vi "Excel___Adjust Main Page.vi"(0 "Cells Ref In":refnum<k7>, 1 "Standards Used":string[][](array[string]), 2 "Standards Count":i32, 3 "Machine Specs":string[][](array[string]), 4 "Specs Count":i32, 5 "Error In":errorcluster, 9 "Too Many?":bool) -> (14 "Cells Ref Out":refnum<k7>, 19 "Error Out":errorcluster)   [LabVIEW 2013]
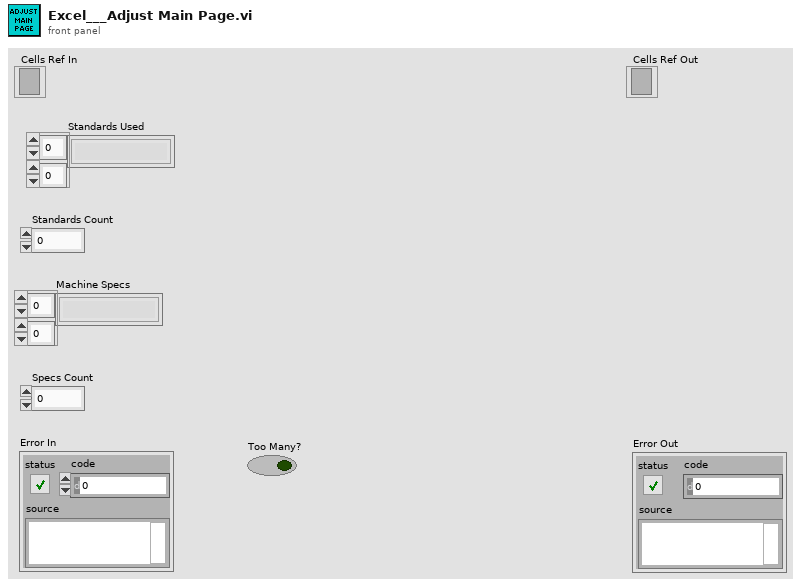
[diagram p1: front panel]
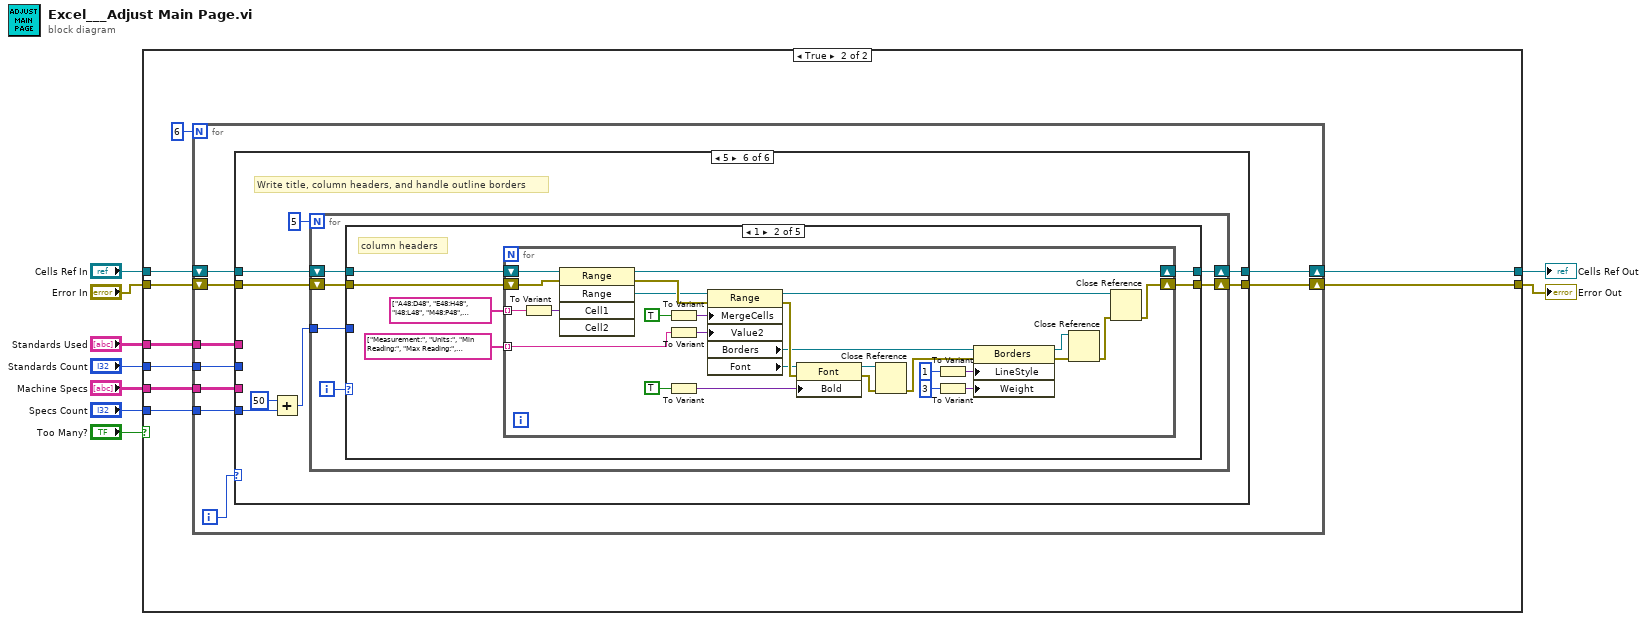
[diagram p0: block diagram]
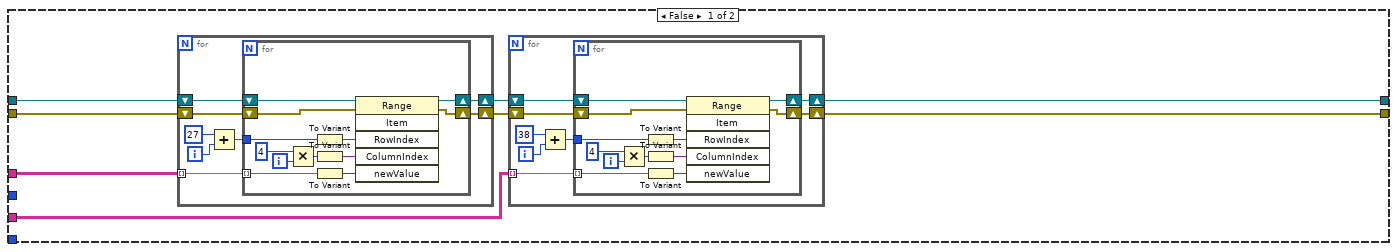
[diagram p2: hidden frame]
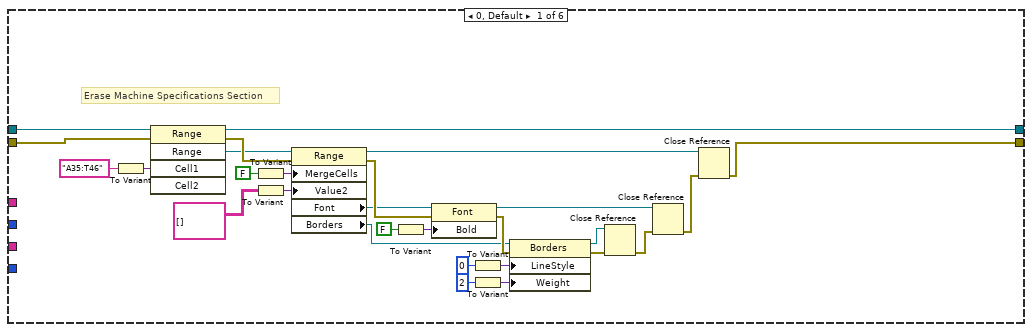
[diagram p3: hidden frame]
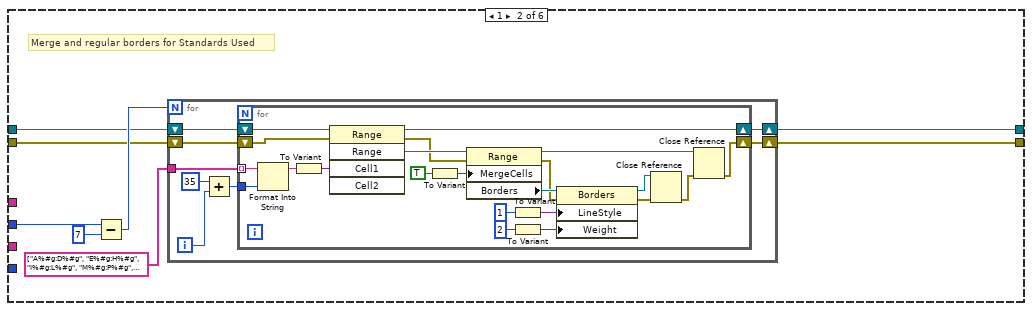
[diagram p4: hidden frame]
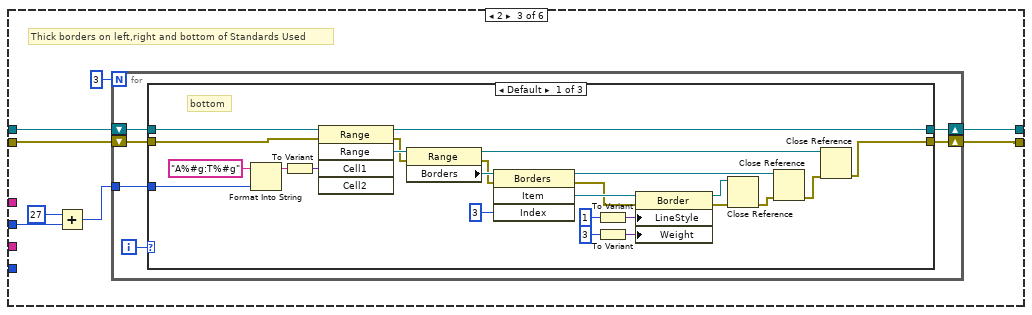
[diagram p5: hidden frame]
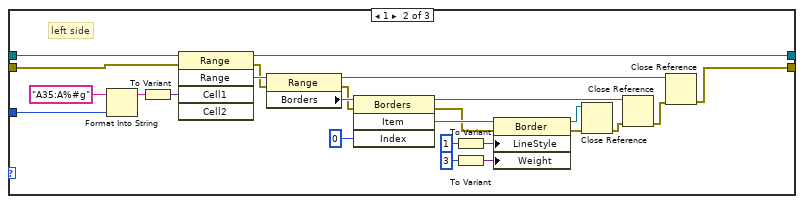
[diagram p6: hidden frame]
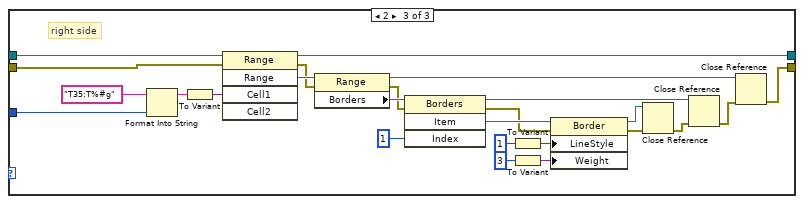
[diagram p7: hidden frame]
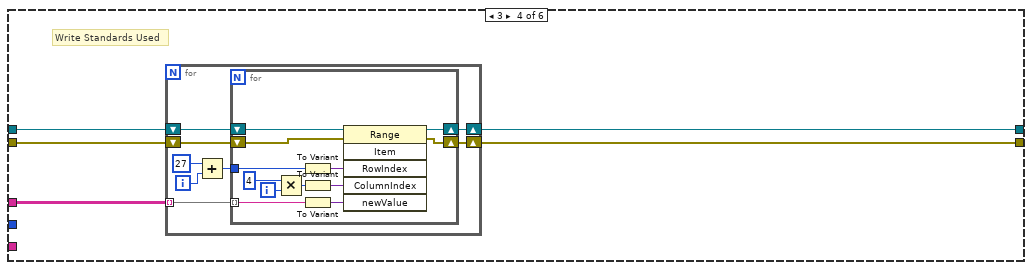
[diagram p8: hidden frame]
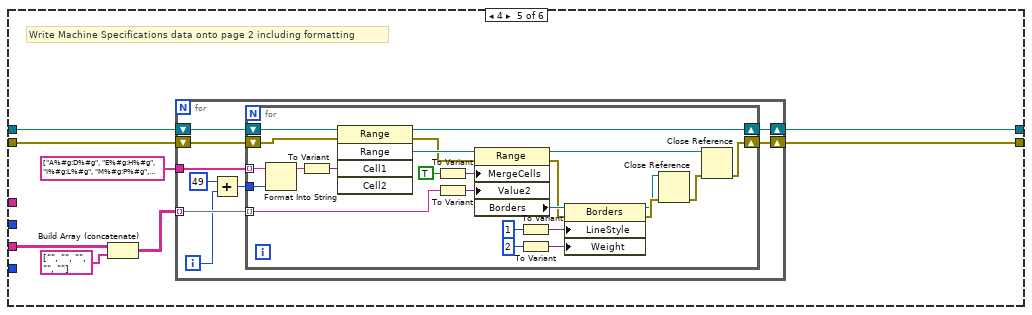
[diagram p9: hidden frame]
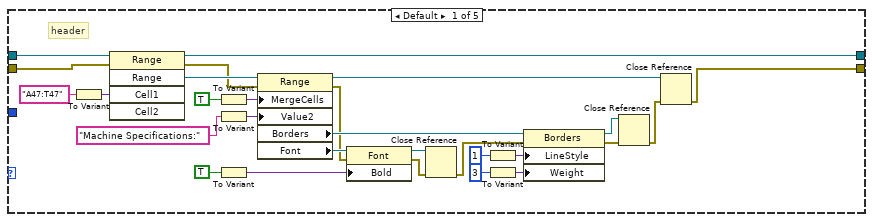
[diagram p10: hidden frame]
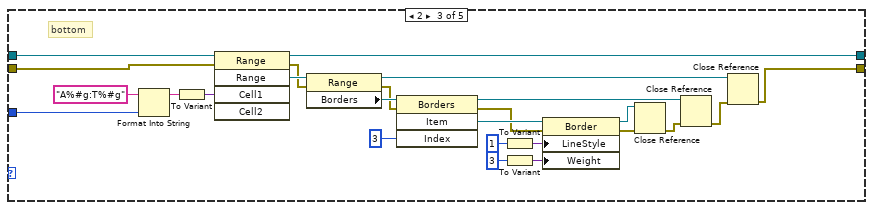
[diagram p11: hidden frame]
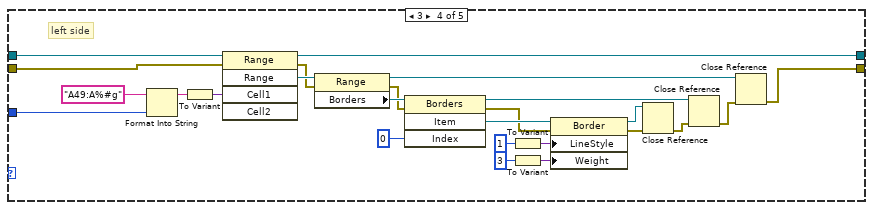
[diagram p12: hidden frame]
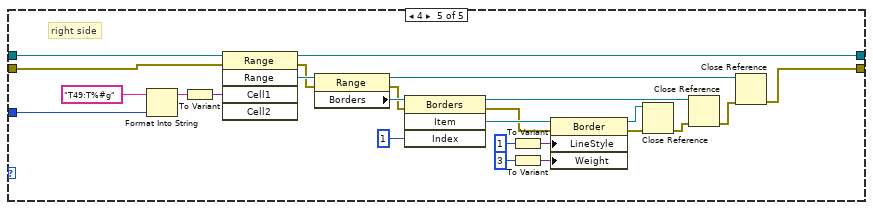
[diagram p13: hidden frame]
diagram:
  n1 = case shown="True" "Too Many?" {
    tunnel: "Error In" -> [w17 w65]
    tunnel: "Standards Used" -> [w16 w64]
    tunnel: "Cells Ref In" -> [w14 w66]
    tunnel: [w13 w61] -> w4
    tunnel: [w12 w62] -> w3
    tunnel: "Machine Specs" -> [w10 w63]
    tunnel: "Standards Count" -> [_ w60]
    tunnel: "Specs Count" -> [_ w59]
    frame False {
      n2 = for {
        shift-right: [w23] -> w11
        shift-left: w14 -> [w25]
        shift-right: [w22] -> w15
        shift-left: w17 -> [w24]
        tunnel: w16 -> [w21] mode=indexing
        i -> [w20]
        n3 = Add(x=27, y=w20) -> (x+y=w18:i32)
        n4 = for {
          shift-right: [w35] -> w23
          shift-left: w25 -> [w37]
          shift-right: [w32] -> w22
          shift-left: w24 -> [w36]
          tunnel: w21 -> [w34] mode=indexing
          tunnel: w18 -> [w29]
          i -> [w28]
          n5 = Multiply(x=4, y=w28) -> (x*y=w26:i32)
          n6 = To Variant(anything=w29) -> (Variant=w31:variant)
          n7 = To Variant(anything=w26) -> (Variant=w30:variant)
          n8 = To Variant(anything=w34) -> (Variant=w33:variant)
          n9 = invoke class="Range" method="Item"(reference=w37, error in=w36, "RowIndex"=w31, "ColumnIndex"=w30, "newValue"=w33) -> (reference out=w35:refnum<k7>, error out=w32:errorcluster)  [unwired: 1 in, 4 out]
        }
      }
      n10 = for {
        shift-right: [w43] -> w13
        shift-left: w11 -> [w45]
        shift-right: [w42] -> w12
        shift-left: w15 -> [w44]
        tunnel: w10 -> [w41] mode=indexing
        i -> [w40]
        n11 = Add(x=38, y=w40) -> (x+y=w38:i32)
        n12 = for {
          shift-right: [w55] -> w43
          shift-left: w45 -> [w57]
          shift-right: [w52] -> w42
          shift-left: w44 -> [w56]
          tunnel: w41 -> [w54] mode=indexing
          tunnel: w38 -> [w49]
          i -> [w48]
          n13 = Multiply(x=4, y=w48) -> (x*y=w46:i32)
          n14 = To Variant(anything=w49) -> (Variant=w51:variant)
          n15 = To Variant(anything=w46) -> (Variant=w50:variant)
          n16 = To Variant(anything=w54) -> (Variant=w53:variant)
          n17 = invoke class="Range" method="Item"(reference=w57, error in=w56, "RowIndex"=w51, "ColumnIndex"=w50, "newValue"=w53) -> (reference out=w55:refnum<k7>, error out=w52:errorcluster)  [unwired: 1 in, 4 out]
        }
      }
    }
    frame True {
      n18 = for {
        N: 6 -> [_]
        tunnel: w64 -> [w73]
        tunnel: w63 -> [w72]
        shift-right: [w70] -> w61
        shift-left: w66 -> [w75]
        shift-right: [w71] -> w62
        shift-left: w65 -> [w74]
        tunnel: w60 -> [w68]
        tunnel: w59 -> [w67]
        i -> [w69]
        n19 = case shown="5" w69 {
          tunnel: w75 -> [w79 w107 w149 w235 w262 w303]
          tunnel: w74 -> [w78 w106 w148 w234 w261 w302]
          tunnel: w73 -> [_ _ _ w233 _ _]
          tunnel: w72 -> [_ _ _ _ w260 _]
          tunnel: [w77 w105 w146 w232 w257 w301] -> w70
          tunnel: [w76 w104 w145 w231 w256 w300] -> w71
          tunnel: w68 -> [_ w110 w144 _ _ _]
          tunnel: w67 -> [_ _ _ _ _ w299]
          frame 0, Default {
            # "Erase Machine Specifications Section"
            n20 = To Variant(anything="A35:T46") -> (Variant=w80:variant)
            n21 = invoke class="Range" method="Range"(reference=w79, error in=w78, "Cell1"=w80) -> (reference out=w77:refnum<k7>, error out=w96:errorcluster, "Range"=w82:refnum<k7>)  [unwired: 2 in, 2 out]
            n22 = To Variant(anything=FALSE) -> (Variant=w83:variant)
            n23 = To Variant(anything=string[][] []) -> (Variant=w86:variant)
            n24 = property class="Range"(reference=w82, error in=w96, "MergeCells"=w83, "Value2"=w86) -> (reference out=w102:refnum<k7>, error out=w97:errorcluster, "Font"=w85:refnum<k7>, "Borders"=w88:refnum<k7>)
            n25 = To Variant(anything=FALSE) -> (Variant=w94:variant)
            n26 = property class="Font"(reference=w85, error in=w97, "Bold"=w94) -> (reference out=w101:refnum<k7>, error out=w95:errorcluster)
            n27 = To Variant(anything=0) -> (Variant=w89:variant)
            n28 = To Variant(anything=2) -> (Variant=w90:variant)
            n29 = property class="Borders"(reference=w88, error in=w95, "LineStyle"=w89, "Weight"=w90) -> (reference out=w99:refnum<k7>, error out=w98:errorcluster)
            n30 = Close Reference(reference=w99, error in (no error)=w98) -> (error out=w100:errorcluster)
            n31 = Close Reference(reference=w101, error in (no error)=w100) -> (error out=w103:errorcluster)
            n32 = Close Reference(reference=w102, error in (no error)=w103) -> (error out=w76:errorcluster)
          }
          frame 1 {
            # "Merge and regular borders for Standards Used"
            n33 = Subtract(x=w110, y=7) -> (x-y=w108:i32)
            n34 = for {
              N: w108 -> [_]
              tunnel: string[] ["A%#g:D%#g", "E%#g:H%#g", "I%#g:L%#g", "M%#g:P%#g", "Q%#g:T%#g"] -> [w119]
              shift-right: [w114] -> w105
              shift-left: w107 -> [w116]
              shift-right: [w113] -> w104
              shift-left: w106 -> [w117]
              i -> [w112]
              n35 = Add(x=35, y=w112) -> (x+y=w115:i32)
              n36 = for {
                tunnel: w119 -> [w141] mode=indexing
                tunnel: w115 -> [w140]
                shift-right: [w122] -> w113
                shift-left: w117 -> [w137]
                shift-right: [w120] -> w114
                shift-left: w116 -> [w136]
                n37 = Format Into String(initial string=w141, w140) -> (resulting string=w139:string)  [unwired: 2 in, 1 out]
                n38 = To Variant(anything=w139) -> (Variant=w138:variant)
                n39 = invoke class="Range" method="Range"(reference=w136, error in=w137, "Cell1"=w138) -> (reference out=w120:refnum<k7>, error out=w132:errorcluster, "Range"=w133:refnum<k7>)  [unwired: 2 in, 2 out]
                n40 = To Variant(anything=TRUE) -> (Variant=w134:variant)
                n41 = property class="Range"(reference=w133, error in=w132, "MergeCells"=w134) -> (reference out=w121:refnum<k7>, error out=w126:errorcluster, "Borders"=w131:refnum<k7>)
                n42 = To Variant(anything=1) -> (Variant=w128:variant)
                n43 = To Variant(anything=2) -> (Variant=w127:variant)
                n44 = property class="Borders"(reference=w131, error in=w126, "LineStyle"=w128, "Weight"=w127) -> (reference out=w124:refnum<k7>, error out=w125:errorcluster)
                n45 = Close Reference(reference=w124, error in (no error)=w125) -> (error out=w123:errorcluster)
                n46 = Close Reference(reference=w121, error in (no error)=w123) -> (error out=w122:errorcluster)
              }
            }
          }
          frame 2 {
            # "Thick borders on left,right and bottom of Standards Used"
            n47 = Add(x=27, y=w144) -> (x+y=w142:i32)
            n48 = for {
              N: 3 -> [_]
              shift-right: [w155] -> w146
              shift-left: w149 -> [w153]
              tunnel: w142 -> [w154]
              shift-right: [w152] -> w145
              shift-left: w148 -> [w151]
              i -> [w150]
              n49 = case shown="Default" w150 {
                tunnel: [w180 w203 w228] -> w155
                tunnel: w154 -> [w156 w181 w206]
                tunnel: w153 -> [w179 w201 w226]
                tunnel: [w178 w191 w216] -> w152
                tunnel: w151 -> [w177 w190 w215]
                frame Default {
                  # "bottom"
                  n50 = Format Into String(initial string="A%#g:T%#g", w156) -> (resulting string=w176:string)  [unwired: 2 in, 1 out]
                  n51 = To Variant(anything=w176) -> (Variant=w175:variant)
                  n52 = invoke class="Range" method="Range"(reference=w179, error in=w177, "Cell1"=w175) -> (reference out=w180:refnum<k7>, error out=w165:errorcluster, "Range"=w173:refnum<k7>)  [unwired: 2 in, 2 out]
                  n53 = property class="Range"(reference=w173, error in=w165) -> (reference out=w166:refnum<k7>, error out=w162:errorcluster, "Borders"=w164:refnum<k7>)
                  n54 = invoke class="Borders" method="Item"(reference=w164, error in=w162, "Index"=3) -> (reference out=w159:refnum<k7>, error out=w157:errorcluster, "Item"=w163:refnum<k7>)  [unwired: 1 in, 1 out]
                  n55 = To Variant(anything=1) -> (Variant=w172:variant)
                  n56 = To Variant(anything=3) -> (Variant=w171:variant)
                  n57 = property class="Border"(reference=w163, error in=w157, "LineStyle"=w172, "Weight"=w171) -> (reference out=w167:refnum<k7>, error out=w168:errorcluster)
                  n58 = Close Reference(reference=w167, error in (no error)=w168) -> (error out=w161:errorcluster)
                  n59 = Close Reference(reference=w159, error in (no error)=w161) -> (error out=w160:errorcluster)
                  n60 = Close Reference(reference=w166, error in (no error)=w160) -> (error out=w178:errorcluster)
                }
                frame 1 {
                  # "left side"
                  n61 = Format Into String(initial string="A35:A%#g", w181) -> (resulting string=w205:string)  [unwired: 2 in, 1 out]
                  n62 = To Variant(anything=w205) -> (Variant=w204:variant)
                  n63 = invoke class="Range" method="Range"(reference=w201, error in=w190, "Cell1"=w204) -> (reference out=w203:refnum<k7>, error out=w192:errorcluster, "Range"=w200:refnum<k7>)  [unwired: 2 in, 2 out]
                  n64 = property class="Range"(reference=w200, error in=w192) -> (reference out=w193:refnum<k7>, error out=w187:errorcluster, "Borders"=w189:refnum<k7>)
                  n65 = invoke class="Borders" method="Item"(reference=w189, error in=w187, "Index"=0) -> (reference out=w184:refnum<k7>, error out=w182:errorcluster, "Item"=w188:refnum<k7>)  [unwired: 1 in, 1 out]
                  n66 = To Variant(anything=1) -> (Variant=w199:variant)
                  n67 = To Variant(anything=3) -> (Variant=w198:variant)
                  n68 = property class="Border"(reference=w188, error in=w182, "LineStyle"=w199, "Weight"=w198) -> (reference out=w194:refnum<k7>, error out=w195:errorcluster)
                  n69 = Close Reference(reference=w194, error in (no error)=w195) -> (error out=w186:errorcluster)
                  n70 = Close Reference(reference=w184, error in (no error)=w186) -> (error out=w185:errorcluster)
                  n71 = Close Reference(reference=w193, error in (no error)=w185) -> (error out=w191:errorcluster)
                }
                frame 2 {
                  # "right side"
                  n72 = Format Into String(initial string="T35:T%#g", w206) -> (resulting string=w230:string)  [unwired: 2 in, 1 out]
                  n73 = To Variant(anything=w230) -> (Variant=w229:variant)
                  n74 = invoke class="Range" method="Range"(reference=w226, error in=w215, "Cell1"=w229) -> (reference out=w228:refnum<k7>, error out=w217:errorcluster, "Range"=w225:refnum<k7>)  [unwired: 2 in, 2 out]
                  n75 = property class="Range"(reference=w225, error in=w217) -> (reference out=w218:refnum<k7>, error out=w212:errorcluster, "Borders"=w214:refnum<k7>)
                  n76 = invoke class="Borders" method="Item"(reference=w214, error in=w212, "Index"=1) -> (reference out=w209:refnum<k7>, error out=w207:errorcluster, "Item"=w213:refnum<k7>)  [unwired: 1 in, 1 out]
                  n77 = To Variant(anything=1) -> (Variant=w224:variant)
                  n78 = To Variant(anything=3) -> (Variant=w223:variant)
                  n79 = property class="Border"(reference=w213, error in=w207, "LineStyle"=w224, "Weight"=w223) -> (reference out=w219:refnum<k7>, error out=w220:errorcluster)
                  n80 = Close Reference(reference=w219, error in (no error)=w220) -> (error out=w211:errorcluster)
                  n81 = Close Reference(reference=w209, error in (no error)=w211) -> (error out=w210:errorcluster)
                  n82 = Close Reference(reference=w218, error in (no error)=w210) -> (error out=w216:errorcluster)
                }
              }
            }
          }
          frame 3 {
            # "Write Standards Used"
            n83 = for {
              shift-right: [w241] -> w232
              shift-left: w235 -> [w243]
              shift-right: [w240] -> w231
              shift-left: w234 -> [w242]
              tunnel: w233 -> [w239] mode=indexing
              i -> [w238]
              n84 = Add(x=27, y=w238) -> (x+y=w236:i32)
              n85 = for {
                shift-right: [w253] -> w241
                shift-left: w243 -> [w255]
                shift-right: [w250] -> w240
                shift-left: w242 -> [w254]
                tunnel: w239 -> [w252] mode=indexing
                tunnel: w236 -> [w247]
                i -> [w246]
                n86 = Multiply(x=4, y=w246) -> (x*y=w244:i32)
                n87 = To Variant(anything=w247) -> (Variant=w249:variant)
                n88 = To Variant(anything=w244) -> (Variant=w248:variant)
                n89 = To Variant(anything=w252) -> (Variant=w251:variant)
                n90 = invoke class="Range" method="Item"(reference=w255, error in=w254, "RowIndex"=w249, "ColumnIndex"=w248, "newValue"=w251) -> (reference out=w253:refnum<k7>, error out=w250:errorcluster)  [unwired: 1 in, 4 out]
              }
            }
          }
          frame 4 {
            # "Write Machine Specifications data onto page 2 including formatting"
            n91 = Build Array (concatenate)(w260, string[] ["", "", "", "", ""]) -> (w258:string[][])
            n92 = for {
              tunnel: string[] ["A%#g:D%#g", "E%#g:H%#g", "I%#g:L%#g", "M%#g:P%#g", "Q%#g:T%#g"] -> [w272]
              shift-right: [w267] -> w257
              shift-left: w262 -> [w269]
              shift-right: [w266] -> w256
              shift-left: w261 -> [w270]
              tunnel: w258 -> [w265] mode=indexing
              i -> [w264]
              n93 = Add(x=49, y=w264) -> (x+y=w268:i32)
              n94 = for {
                tunnel: w272 -> [w296] mode=indexing
                tunnel: w268 -> [w295]
                shift-right: [w277] -> w266
                shift-left: w270 -> [w292]
                shift-right: [w275] -> w267
                shift-left: w269 -> [w291]
                tunnel: w265 -> [w274] mode=indexing
                n95 = Format Into String(initial string=w296, w295) -> (resulting string=w294:string)  [unwired: 2 in, 1 out]
                n96 = To Variant(anything=w294) -> (Variant=w293:variant)
                n97 = invoke class="Range" method="Range"(reference=w291, error in=w292, "Cell1"=w293) -> (reference out=w275:refnum<k7>, error out=w287:errorcluster, "Range"=w288:refnum<k7>)  [unwired: 2 in, 2 out]
                n98 = To Variant(anything=TRUE) -> (Variant=w289:variant)
                n99 = To Variant(anything=w274) -> (Variant=w273:variant)
                n100 = property class="Range"(reference=w288, error in=w287, "MergeCells"=w289, "Value2"=w273) -> (reference out=w276:refnum<k7>, error out=w281:errorcluster, "Borders"=w286:refnum<k7>)
                n101 = To Variant(anything=1) -> (Variant=w283:variant)
                n102 = To Variant(anything=2) -> (Variant=w282:variant)
                n103 = property class="Borders"(reference=w286, error in=w281, "LineStyle"=w283, "Weight"=w282) -> (reference out=w279:refnum<k7>, error out=w280:errorcluster)
                n104 = Close Reference(reference=w279, error in (no error)=w280) -> (error out=w278:errorcluster)
                n105 = Close Reference(reference=w276, error in (no error)=w278) -> (error out=w277:errorcluster)
              }
            }
          }
          frame 5 {
            # "Write title, column headers, and handle outline borders"
            n106 = Add(x=50, y=w299) -> (x+y=w297:i32)
            n107 = for {
              N: 5 -> [_]
              shift-right: [w310] -> w301
              shift-left: w303 -> [w308]
              tunnel: w297 -> [w309]
              shift-right: [w307] -> w300
              shift-left: w302 -> [w306]
              i -> [w305]
              n108 = case shown="1" w305 {
                tunnel: [w337 w342 w397 w420 w445] -> w310
                tunnel: w309 -> [_ _ w373 w398 w423]
                tunnel: w308 -> [w336 w344 w396 w418 w443]
                tunnel: [w325 w341 w395 w408 w433] -> w307
                tunnel: w306 -> [w324 w343 w394 w407 w432]
                frame Default {
                  # "header"
                  n109 = To Variant(anything="A47:T47") -> (Variant=w338:variant)
                  n110 = invoke class="Range" method="Range"(reference=w336, error in=w324, "Cell1"=w338) -> (reference out=w337:refnum<k7>, error out=w326:errorcluster, "Range"=w335:refnum<k7>)  [unwired: 2 in, 2 out]
                  n111 = To Variant(anything=TRUE) -> (Variant=w315:variant)
                  n112 = To Variant(anything="Machine Specifications:") -> (Variant=w314:variant)
                  n113 = To Variant(anything=TRUE) -> (Variant=w311:variant)
                  n114 = property class="Range"(reference=w335, error in=w326, "MergeCells"=w315, "Value2"=w314) -> (reference out=w327:refnum<k7>, error out=w321:errorcluster, "Borders"=w334:refnum<k7>, "Font"=w322:refnum<k7>)
                  n115 = property class="Font"(reference=w322, error in=w321, "Bold"=w311) -> (reference out=w320:refnum<k7>, error out=w319:errorcluster)
                  n116 = Close Reference(reference=w320, error in (no error)=w319) -> (error out=w318:errorcluster)
                  n117 = To Variant(anything=1) -> (Variant=w333:variant)
                  n118 = To Variant(anything=3) -> (Variant=w332:variant)
                  n119 = property class="Borders"(reference=w334, error in=w318, "LineStyle"=w333, "Weight"=w332) -> (reference out=w328:refnum<k7>, error out=w329:errorcluster)
                  n120 = Close Reference(reference=w328, error in (no error)=w329) -> (error out=w317:errorcluster)
                  n121 = Close Reference(reference=w327, error in (no error)=w317) -> (error out=w325:errorcluster)
                }
                frame 1 {
                  # "column headers"
                  n122 = for {
                    shift-right: [w348] -> w341
                    shift-left: w343 -> [w349]
                    shift-right: [w347] -> w342
                    shift-left: w344 -> [w350]
                    tunnel: string[] ["A48:D48", "E48:H48", "I48:L48", "M48:P48", "Q48:T48"] -> [w346] mode=indexing
                    tunnel: string[] ["Measurement:", "Units:", "Min Reading:", "Max Reading:", "Tolerance:"] -> [w345] mode=indexing
                    n123 = To Variant(anything=w346) -> (Variant=w351:variant)
                    n124 = invoke class="Range" method="Range"(reference=w350, error in=w349, "Cell1"=w351) -> (reference out=w347:refnum<k7>, error out=w361:errorcluster, "Range"=w352:refnum<k7>)  [unwired: 2 in, 2 out]
                    n125 = To Variant(anything=TRUE) -> (Variant=w369:variant)
                    n126 = To Variant(anything=w345) -> (Variant=w370:variant)
                    n127 = To Variant(anything=TRUE) -> (Variant=w372:variant)
                    n128 = property class="Range"(reference=w352, error in=w361, "MergeCells"=w369, "Value2"=w370) -> (reference out=w360:refnum<k7>, error out=w363:errorcluster, "Borders"=w353:refnum<k7>, "Font"=w362:refnum<k7>)
                    n129 = property class="Font"(reference=w362, error in=w363, "Bold"=w372) -> (reference out=w364:refnum<k7>, error out=w365:errorcluster)
                    n130 = Close Reference(reference=w364, error in (no error)=w365) -> (error out=w366:errorcluster)
                    n131 = To Variant(anything=1) -> (Variant=w354:variant)
                    n132 = To Variant(anything=3) -> (Variant=w355:variant)
                    n133 = property class="Borders"(reference=w353, error in=w366, "LineStyle"=w354, "Weight"=w355) -> (reference out=w359:refnum<k7>, error out=w358:errorcluster)
                    n134 = Close Reference(reference=w359, error in (no error)=w358) -> (error out=w367:errorcluster)
                    n135 = Close Reference(reference=w360, error in (no error)=w367) -> (error out=w348:errorcluster)
                  }
                }
                frame 2 {
                  # "bottom"
                  n136 = Format Into String(initial string="A%#g:T%#g", w373) -> (resulting string=w393:string)  [unwired: 2 in, 1 out]
                  n137 = To Variant(anything=w393) -> (Variant=w392:variant)
                  n138 = invoke class="Range" method="Range"(reference=w396, error in=w394, "Cell1"=w392) -> (reference out=w397:refnum<k7>, error out=w382:errorcluster, "Range"=w390:refnum<k7>)  [unwired: 2 in, 2 out]
                  n139 = property class="Range"(reference=w390, error in=w382) -> (reference out=w383:refnum<k7>, error out=w379:errorcluster, "Borders"=w381:refnum<k7>)
                  n140 = invoke class="Borders" method="Item"(reference=w381, error in=w379, "Index"=3) -> (reference out=w376:refnum<k7>, error out=w374:errorcluster, "Item"=w380:refnum<k7>)  [unwired: 1 in, 1 out]
                  n141 = To Variant(anything=1) -> (Variant=w389:variant)
                  n142 = To Variant(anything=3) -> (Variant=w388:variant)
                  n143 = property class="Border"(reference=w380, error in=w374, "LineStyle"=w389, "Weight"=w388) -> (reference out=w384:refnum<k7>, error out=w385:errorcluster)
                  n144 = Close Reference(reference=w384, error in (no error)=w385) -> (error out=w378:errorcluster)
                  n145 = Close Reference(reference=w376, error in (no error)=w378) -> (error out=w377:errorcluster)
                  n146 = Close Reference(reference=w383, error in (no error)=w377) -> (error out=w395:errorcluster)
                }
                frame 3 {
                  # "left side"
                  n147 = Format Into String(initial string="A49:A%#g", w398) -> (resulting string=w422:string)  [unwired: 2 in, 1 out]
                  n148 = To Variant(anything=w422) -> (Variant=w421:variant)
                  n149 = invoke class="Range" method="Range"(reference=w418, error in=w407, "Cell1"=w421) -> (reference out=w420:refnum<k7>, error out=w409:errorcluster, "Range"=w417:refnum<k7>)  [unwired: 2 in, 2 out]
                  n150 = property class="Range"(reference=w417, error in=w409) -> (reference out=w410:refnum<k7>, error out=w404:errorcluster, "Borders"=w406:refnum<k7>)
                  n151 = invoke class="Borders" method="Item"(reference=w406, error in=w404, "Index"=0) -> (reference out=w401:refnum<k7>, error out=w399:errorcluster, "Item"=w405:refnum<k7>)  [unwired: 1 in, 1 out]
                  n152 = To Variant(anything=1) -> (Variant=w416:variant)
                  n153 = To Variant(anything=3) -> (Variant=w415:variant)
                  n154 = property class="Border"(reference=w405, error in=w399, "LineStyle"=w416, "Weight"=w415) -> (reference out=w411:refnum<k7>, error out=w412:errorcluster)
                  n155 = Close Reference(reference=w411, error in (no error)=w412) -> (error out=w403:errorcluster)
                  n156 = Close Reference(reference=w401, error in (no error)=w403) -> (error out=w402:errorcluster)
                  n157 = Close Reference(reference=w410, error in (no error)=w402) -> (error out=w408:errorcluster)
                }
                frame 4 {
                  # "right side"
                  n158 = Format Into String(initial string="T49:T%#g", w423) -> (resulting string=w447:string)  [unwired: 2 in, 1 out]
                  n159 = To Variant(anything=w447) -> (Variant=w446:variant)
                  n160 = invoke class="Range" method="Range"(reference=w443, error in=w432, "Cell1"=w446) -> (reference out=w445:refnum<k7>, error out=w434:errorcluster, "Range"=w442:refnum<k7>)  [unwired: 2 in, 2 out]
                  n161 = property class="Range"(reference=w442, error in=w434) -> (reference out=w435:refnum<k7>, error out=w429:errorcluster, "Borders"=w431:refnum<k7>)
                  n162 = invoke class="Borders" method="Item"(reference=w431, error in=w429, "Index"=1) -> (reference out=w426:refnum<k7>, error out=w424:errorcluster, "Item"=w430:refnum<k7>)  [unwired: 1 in, 1 out]
                  n163 = To Variant(anything=1) -> (Variant=w441:variant)
                  n164 = To Variant(anything=3) -> (Variant=w440:variant)
                  n165 = property class="Border"(reference=w430, error in=w424, "LineStyle"=w441, "Weight"=w440) -> (reference out=w436:refnum<k7>, error out=w437:errorcluster)
                  n166 = Close Reference(reference=w436, error in (no error)=w437) -> (error out=w428:errorcluster)
                  n167 = Close Reference(reference=w426, error in (no error)=w428) -> (error out=w427:errorcluster)
                  n168 = Close Reference(reference=w435, error in (no error)=w427) -> (error out=w433:errorcluster)
                }
              }
            }
          }
        }
      }
    }
  }
  "Cells Ref Out" <- w4
  "Error Out" <- w3
